vi "IP Server Check.vi"(11 "IP Address":string) -> (3 "IP Same as execution Computer?":bool)   [LabVIEW 2011]
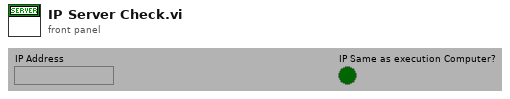
[diagram p1: front panel]
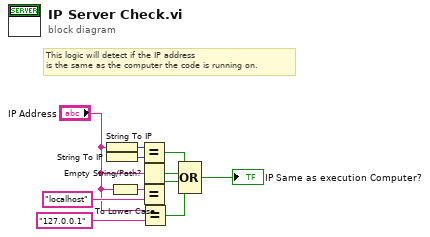
[diagram p0: block diagram]
diagram:
  # "This logic will detect if the IP address \nis the same as the computer the code is running on."
  n1 = String To IP(1:"IP Address") -> (0:w9:u32)
  n2 = String To IP() -> (0:w8:u32)  [unwired: 1 out]
  n3 = To Lower Case(string="IP Address") -> (all lower case string=w10:string)
  n4 = Equal?(x=w9, y=w8) -> (x = y?=w7:bool)
  n5 = Empty String/Path?(string/path="IP Address") -> (empty?=w6:bool)
  n6 = Equal?(x=w10, y="localhost") -> (x = y?=w5:bool)
  n7 = Equal?(x="IP Address", y="127.0.0.1") -> (x = y?=w4:bool)
  n8 = Compound Arithmetic op=OR(w7, w6, w5, w4) -> (→"IP Same as execution Computer?":bool)
